vi "FromMagnitudeToImpedance (SubVI).vi"(2 "GainFactor":dbl[](array[numeric])=[1.5759e-10], 3 "I":dbl[](array[numeric]), 4 "R":dbl[](array[numeric])) -> (0 "Phase":dbl[](array[numeric]), 1 "Impedance":dbl[](array[numeric]))   [LabVIEW 2017]
uses:
  <vilib>/imath/engines/lvmath2/RunTimeEngine/ArithmeticOperatorToken/NIMS_ArithmeticOperator_plus.vi
  <instcachedir>/0/NIMS_ArithmeticOperator_plus_9255C7DA94A9479C92F91DC2DA9A664F.lvgen/NIMS_ArithmeticOperator_plus_9255C7DA94A9479C92F91DC2DA9A664F_004.vi
  <vilib>/imathl/engines/lvmath/Functions/Error Handling/Create Error.vi
  <vilib>/imath/engines/lvmath2/RunTimeEngine/ArithmeticOperatorToken/NIMS_ArithmeticOperator_times.vi
  <instcachedir>/0/NIMS_ArithmeticOperator_times_9BECD6C28351466A83A029AF2762CD58.lvgen/NIMS_ArithmeticOperator_times_9BECD6C28351466A83A029AF2762CD58_000.vi
  <vilib>/imath/engines/lvmath2/RunTimeEngine/ArithmeticOperatorToken/NIMS_ArithmeticOperator_rightdiv.vi
  <instcachedir>/0/NIMS_ArithmeticOperator_rightdiv_EFA95513F40C4B3084B27C9DE6D5A167.lvgen/NIMS_ArithmeticOperator_rightdiv_EFA95513F40C4B3084B27C9DE6D5A167_000.vi
  <vilib>/imath/engines/lvmath2/RunTimeEngine/NodeEndStatement/NIMS_NodeEndStatement_Output.vi
  <instcachedir>/0/NIMS_NodeEndStatement_Output_53EC0D466D134D7ABD903AC30B43404B.lvgen/NIMS_NodeEndStatement_Output_53EC0D466D134D7ABD903AC30B43404B_005.vi
  <vilib>/imath/engines/lvmath2/RunTimeEngine/ErrorHandling/NIMS_Finalize Error.vi
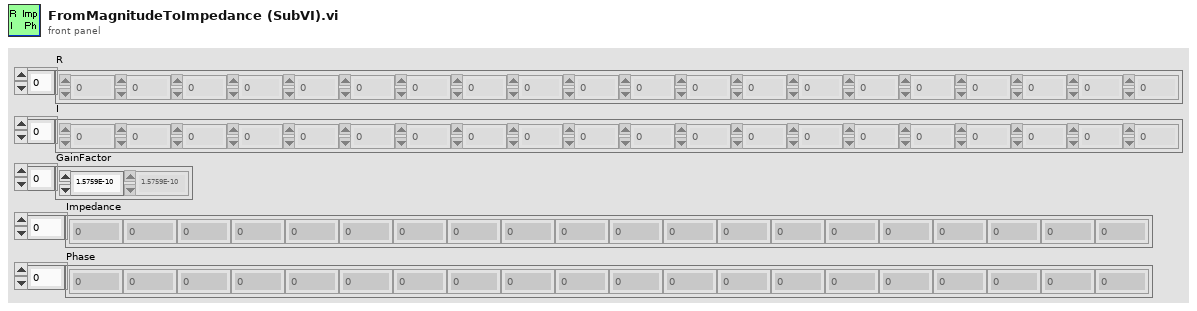
[diagram p1: front panel]
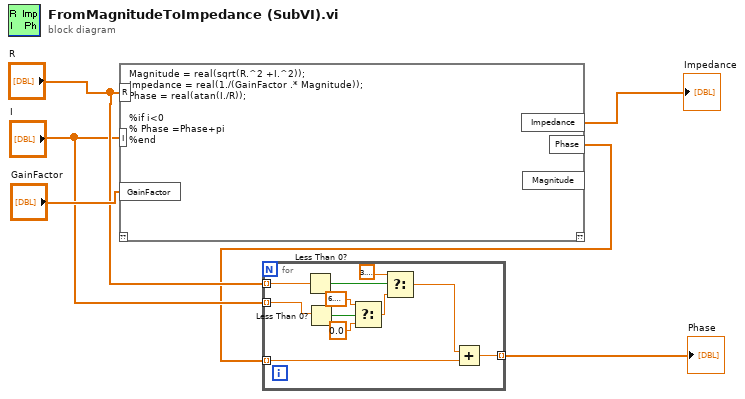
[diagram p0: block diagram]
diagram:
  n1 = mathscript code="Magnitude = real(sqrt(R.^2 +I.^2));\nImpedance = real(1./(GainFactor .* Magnitude));\nPhase = real(atan(I./R));\n\n%if i<0\n% Phase =Phase+pi\n%end"("R"="R", "I"="I", "GainFactor"="GainFactor") -> ("Impedance"=→"Impedance":dbl[], "Phase"=w2:dbl[])  [unwired: 1 in, 2 out]
  n2 = for {
    tunnel: "R" -> [w17] mode=indexing
    tunnel: "I" -> [w15] mode=indexing
    tunnel: w2 -> [w9] mode=indexing
    tunnel: [w7] -> w1 mode=indexing
    n3 = Less Than 0?(x=w17) -> (x < 0?=w16:bool)
    n4 = Less Than 0?(x=w15) -> (x < 0?=w14:bool)
    n5 = Select(t=6.283185307179586, s=w14, f=0.0) -> (s? t:f=w12:dbl)
    n6 = Select(t=3.141592653589793, s=w16, f=w12) -> (s? t:f=w8:dbl)
    n7 = Add(x=w8, y=w9) -> (x+y=w7:dbl)
  }
  "Phase" <- w1
